vi "ROSUnregister.vi"(2 "Err in":path, 4 "Server ROS":T3={"topic port"=0, "Node"="", "topic"="", "type"="", "node port"=0, "error "={"status"=FALSE, "code"=0, "source"=""}, "Direction"=enum."Node", "APIs"=[], "Update (ms)"=1, "write queue"=1}) -> (0 "Err out":path, 1 "Log":T2)   [LabVIEW 2012]
uses:
  <userlib>/ROSforLV/ROS/Code/SubVIs/_ROSControl.ctl
  <userlib>/ROSforLV/ROS/Code/SubVIs/_ROSDirection.ctl
  <userlib>/ROSforLV/ROS/Code/Console/Servers/ServerSubs/ROSLog.ctl
  <userlib>/ROSforLV/ROS/Code/Console/Servers/ServerSubs/MyState.ctl
panel:
  out "unReply":T1
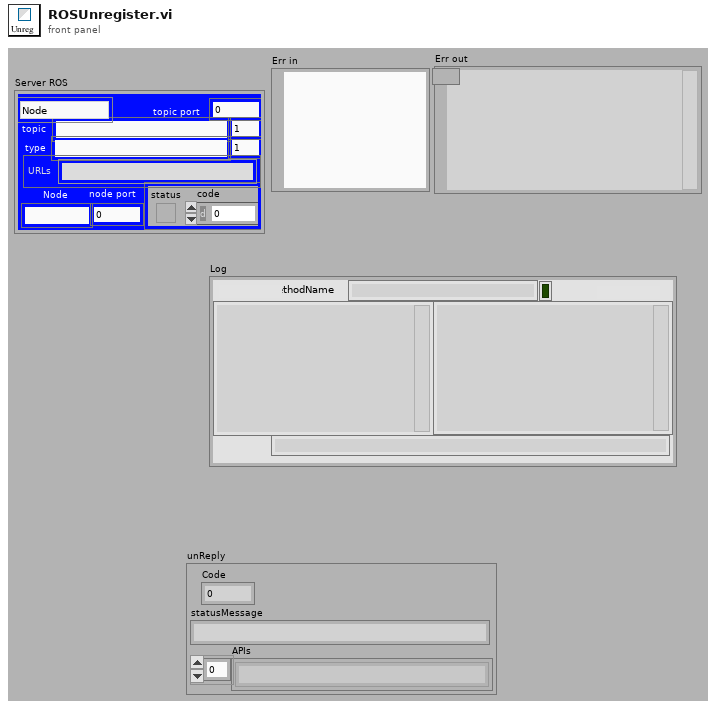
[diagram p1: front panel]
types:
  T1 = cluster{"Code":i8, "statusMessage":string, "APIs":string[]}
  T2 = typedef "ROSLog.ctl" = cluster{"Sent":string, "Reply":string, "MethodName":string, "success":bool, "Dir1":string, "Dir2":string, "Time Stamp":string, "error":errorcluster, "Preamble":string}
  T3 = typedef "_ROSControl.ctl" = cluster{"topic port":u16, "Node":string, "topic":string, "type":string, "node port":u32, "error ":errorcluster, "Direction":T4, "APIs":string[], "Update (ms)":u16, "write queue":u16}
  T4 = typedef "_ROSDirection.ctl" = enum16{"Node", "Publisher", "Subscriber", "Service Client"}
  T5 = typedef "MyState.ctl" = enum16{"No Connection", "Registered", "Connected", "Close"}
  T6 = cluster{"Caller ID":string, "Topic":string, "Caller API":string}
  T7 = enum16{"http://IP:port", "http://IP", "IP:port", "IP only"}
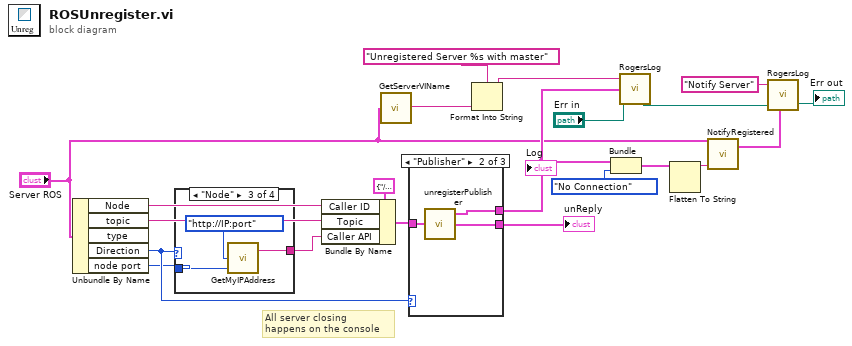
[diagram p0: block diagram]
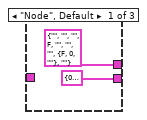
[diagram p2: hidden frame]
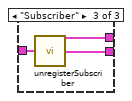
[diagram p3: hidden frame]
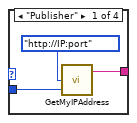
[diagram p4: hidden frame]
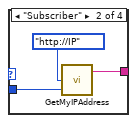
[diagram p5: hidden frame]
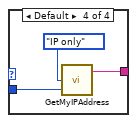
[diagram p6: hidden frame]
diagram:
  # "All server closing\nhappens on the console"
  n1 = Unbundle By Name("Server ROS") -> ("Node"=w16:string, "topic"=w17:string, "Direction"=w18:T4, "node port"=w15:u32)  [unwired: 1 out]
  n2 = case shown="\"Node\"" w18 {
    tunnel: [w24 w27 w30 w33] -> w19
    tunnel: w15 -> [w22 w25 w29 w32]
    frame "Publisher" {
      n3 = call <userlib>:"GetMyIPAddress.vi"("Port"=w22, "Format"=T7."http://IP:port") -> ("URI"=w24:string)  [unwired: 2 in]
    }
    frame "Subscriber" {
      n4 = call <userlib>:"GetMyIPAddress.vi"("Port"=w25, "Format"=T7."http://IP") -> ("URI"=w27:string)  [unwired: 2 in]
    }
    frame "Node" {
      n5 = call <userlib>:"GetMyIPAddress.vi"("Port"=w29, "Format"=T7."http://IP:port") -> ("URI"=w30:string)  [unwired: 2 in]
    }
    frame Default {
      n6 = call <userlib>:"GetMyIPAddress.vi"("Port"=w32, "Format"=T7."IP only") -> ("URI"=w33:string)  [unwired: 2 in]
    }
  }
  n7 = Bundle By Name(cluster=T6 {"Caller ID"="/labview", "Topic"="/topic", "Caller API"="API"} ("Parameters"), "Caller ID"=w16, "Topic"=w17, "Caller API"=w19) -> (w20:T6)
  n8 = call <userlib>:"GetServerVIName.vi"("ROS"="Server ROS") -> ("vi name"=w3:string)
  n9 = case shown="\"Publisher\"" w18 {
    tunnel: w20 -> [_ w38 w41]
    tunnel: [T2 {"Sent"="", "Reply"="", "MethodName"="", "success"=FALSE, "Dir1"="", "Dir2"="", "Time Stamp"="", "error"={"status"=FALSE, "code"=0, "source"=""}, "Preamble"=""} ("Log") w37 w40] -> w9
    tunnel: [T1 {"Code"=0, "statusMessage"="", "APIs"=[]} ("Reply") w36 w39] -> w14
    frame "Node", Default {
    }
    frame "Publisher" {
      n10 = call <userlib>:"unregisterPublisher.vi"("Parameters"=w38) -> ("Reply"=w36:T1, "Log"=w37:T2)  [unwired: 2 in]
    }
    frame "Subscriber" {
      n11 = call <userlib>:"unregisterSubscriber.vi"("Parameters"=w41) -> ("Reply"=w39:T1, "Log"=w40:T2)  [unwired: 2 in]
    }
  }
  "Log" <- w9
  "unReply" <- w14
  n12 = Format Into String(format string="Unregistered Server %s with master" ("Text to add"), w3) -> (resulting string=w1:string)  [unwired: 2 in, 1 out]
  n13 = Bundle("Log"=w9, "MyState"=MyState."No Connection") -> (w13:cluster{"Log":T2, "MyState":T5})  [unwired: 1 in]
  n14 = call <userlib>:"RogersLog.vi"("Text to add"=w1, "Log"=w9, "LogPath in"="Err in") -> ("LogPath out"=w8:path)  [unwired: 2 in, 1 out]
  n15 = Flatten To String(anything=w13) -> (data string=w11:string)  [unwired: 3 in, 2 out]
  n16 = call <userlib>:"NotifyRegistered.vi"("data string"=w11, "ROS"="Server ROS") -> ("ROS out"=w6:T3)  [unwired: 1 in]
  n17 = call <userlib>:"RogersLog.vi"("Text to add"="Notify Server", "ROS"=w6, "LogPath in"=w8) -> ("LogPath out"=→"Err out":path)  [unwired: 2 in, 1 out]
